vi "alternateFrontPanelCommand.vi"(8 "error in (no error)":errorcluster, 11 "TEI9150 in":refnum<class "TEI9150.lvclass">) -> (0 "error out":errorcluster, 1 "Other Item with alternate unit":string, 2 "Current Item with unit":string, 3 "TEI9150 out":refnum<class "TEI9150.lvclass">)   [LabVIEW 2015, in "TEI9150.lvclass"]
uses:
  TEI9150.lvclass
  <userlib>/Common/ILC/ILCModelTypedefs/FinalDelimiter.ctl
  TEI9150.lvclass/TEI9150.ctl
  <userlib>/Common/SerialProtocols/SerialCommunicator/SerialCommunicator.lvclass
  <vilib>/regexp/Match Regular Expression.xnode
  <userlib>/Common/ILC/ILCModelTypedefs/ILCModelTypedefs.lvlib
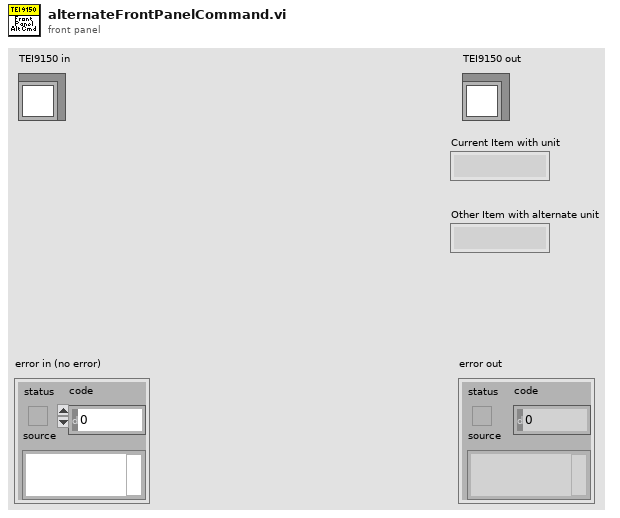
[diagram p1: front panel]
types:
  T1 = typedef "ILCCommon.lvlib/ILCModelTypedefs.lvlib/FinalDelimiter.ctl" = enum16{",", "<CR><LF>"}
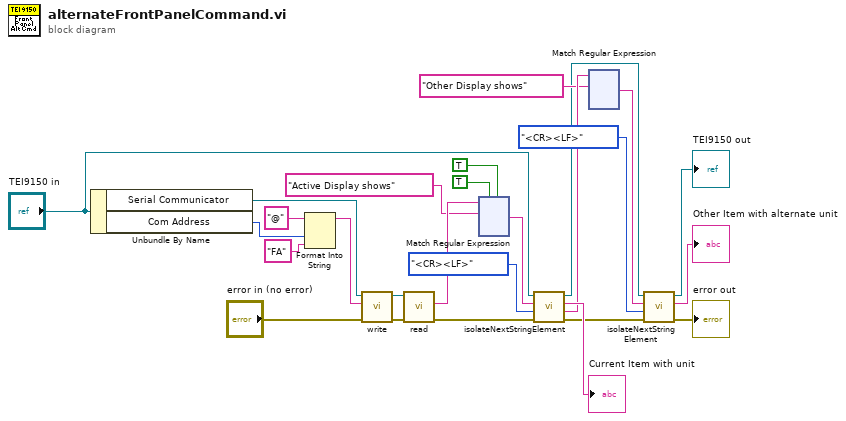
[diagram p0: block diagram]
diagram:
  n1 = Unbundle By Name("TEI9150 in") -> ("Serial Communicator"=w24:refnum<class "SerialCommunicator.lvclass">, "Com Address"=w22:u8)
  n2 = Format Into String(initial string="@", w22, "FA" ("initial string")) -> (resulting string=w20:string)  [unwired: 2 in, 1 out]
  n3 = call-dynamic "write.vi"("error in (no error)"="error in (no error)", "writeString"=w20, "SerialCommunicator in"=w24) -> ("error out"=w26:errorcluster, "SerialCommunicator out"=w25:refnum<class "SerialCommunicator.lvclass">)  [unwired: 7 in]
  n4 = call-dynamic "read.vi"("error in (no error)"=w26, "SerialCommunicator in"=w25) -> ("error out"=w10:errorcluster, "stringRead"=w18:string)  [unwired: 7 in, 1 out]
  n5 = xnode "Match Regular Expression"("input string"=w18, "regular expression"="Active Display shows", "ignore case? (F)"=TRUE, "multiline? (F)"=TRUE) -> ("after match"=w14:string)  [unwired: 2 in, 4 out]
  n6 = call "isolateNextStringElement.vi"("error in (no error)"=w10, "Final Delimiter"=FinalDelimiter."<CR><LF>", "inputString"=w14, "TEI9150 in"="TEI9150 in") -> ("error out"=w2:errorcluster, "remainingString"=w11:string, "extractedSegment"=→"Current Item with unit":string, "TEI9150 out"=w6:refnum<class "TEI9150.lvclass">)  [unwired: 4 in]
  n7 = xnode "Match Regular Expression"("input string"=w11, "regular expression"="Other Display shows") -> ("after match"=w8:string)  [unwired: 4 in, 4 out]
  n8 = call "isolateNextStringElement.vi"("error in (no error)"=w2, "Final Delimiter"=FinalDelimiter."<CR><LF>", "inputString"=w8, "TEI9150 in"=w6) -> ("error out"=→"error out":errorcluster, "extractedSegment"=→"Other Item with alternate unit":string, "TEI9150 out"=→"TEI9150 out":refnum<class "TEI9150.lvclass">)  [unwired: 4 in, 1 out]
